vi "Create Pattern Script(Burst Length).vi"(8 "error in (no error)":errorcluster, 10 "BurstLength":T1, 11 "BML Pattern Creater in":refnum<class "BML Pattern Creater.lvclass">) -> (0 "error out":errorcluster, 2 "String":string, 3 "BML Pattern Creater out":refnum<class "BML Pattern Creater.lvclass">)   [LabVIEW 2018, in "BML Pattern Creater.lvlib" / "BML Pattern Creater.lvclass"]
uses:
  BML Pattern Creater.lvclass
  Ctls/Burst Length.ctl
  Interfaces/Protocol Interface.lvlibp/Interfaces/Protocol Interface/Pin State.ctl
  Interfaces/Protocol Interface.lvlibp/Interfaces/Protocol Interface/Protocol Interface.lvclass
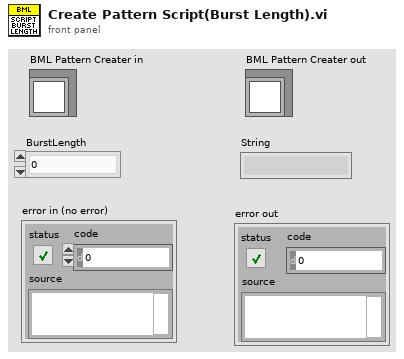
[diagram p1: front panel]
types:
  T1 = typedef "Burst Length.ctl" = enum8{"0", "2", "3", "4", "5", "8", "16", "32"}
  T2 = typedef "Protocol Interface.lvlibp/Protocol Interface.lvclass/Pin State.ctl" = enum16{"0", "1", "L", "H", "X", "V", "D", "M"}
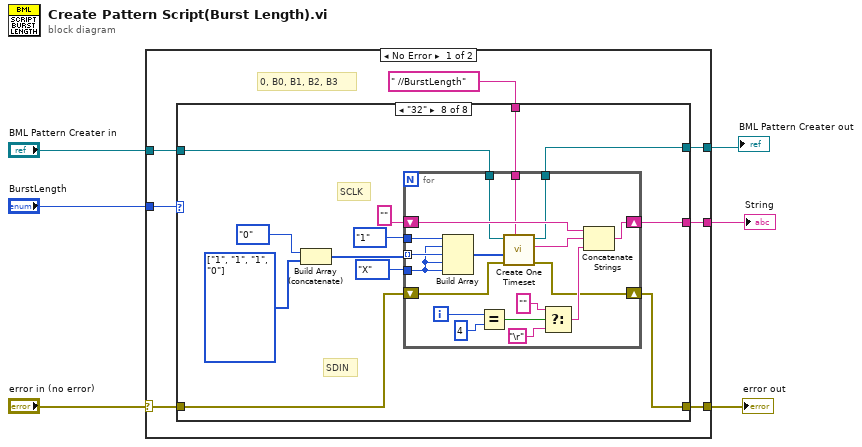
[diagram p0: block diagram]
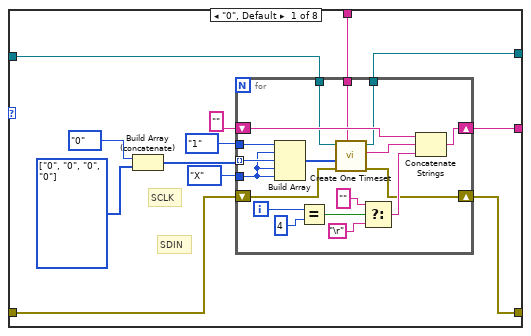
[diagram p2: hidden frame]
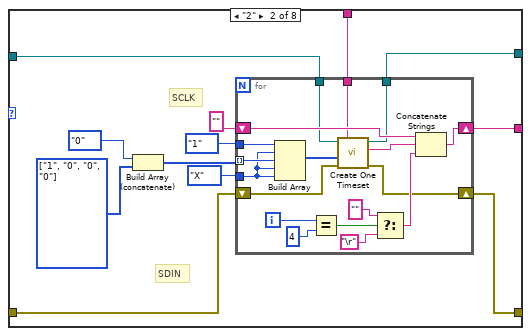
[diagram p3: hidden frame]
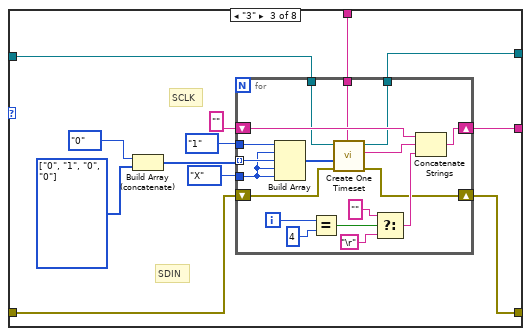
[diagram p4: hidden frame]
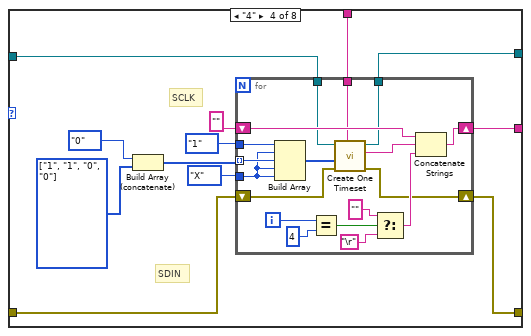
[diagram p5: hidden frame]
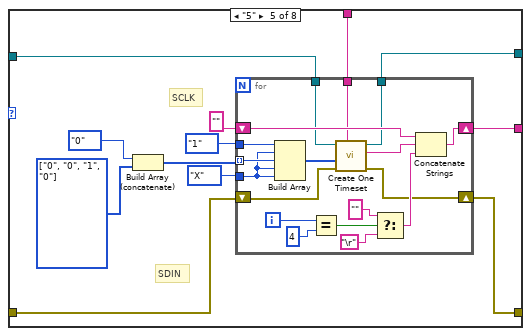
[diagram p6: hidden frame]
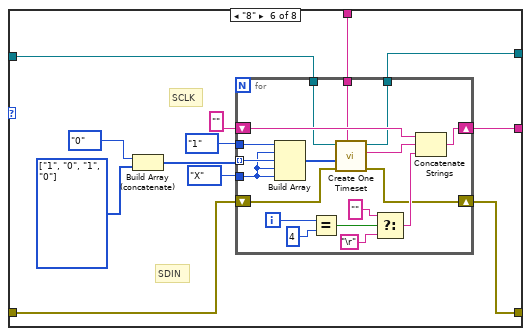
[diagram p7: hidden frame]
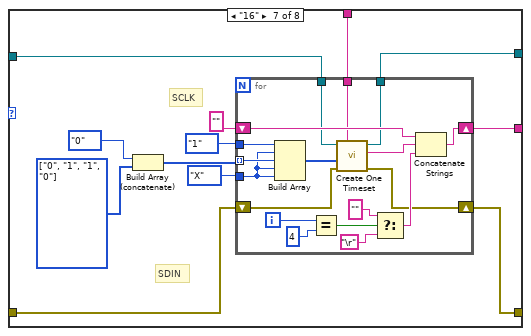
[diagram p8: hidden frame]
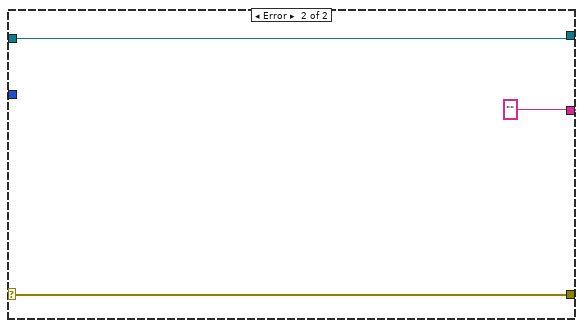
[diagram p9: hidden frame]
diagram:
  n1 = case shown="No Error" "error in (no error)" {
    selector: "error in (no error)" -> [w9 w255]
    tunnel: [w13 ""] -> w5
    tunnel: [w8 w255] -> w4
    tunnel: "BurstLength" -> [w11 _]
    tunnel: "BML Pattern Creater in" -> [w10 w254]
    tunnel: [w7 w254] -> w1
    frame No Error {
      # "0, B0, B1, B2, B3"
      n2 = case shown="\"32\"" w11 {
        tunnel: [w25 w55 w85 w115 w145 w175 w205 w235] -> w13
        tunnel: " //BurstLength" ("Notes") -> [w21 w51 w81 w111 w141 w171 w201 w231]
        tunnel: w10 -> [w17 w47 w77 w107 w137 w167 w197 w227]
        tunnel: [w16 w46 w76 w106 w136 w166 w196 w226] -> w7
        tunnel: w9 -> [w15 w45 w75 w105 w135 w165 w195 w225]
        tunnel: [w14 w44 w74 w104 w134 w164 w194 w224] -> w8
        frame "0", Default {
          w23 = T2[] [enum."0", enum."0", enum."0", enum."0"] items=["0", "1", "L", "H", "X", "V", "D", "M"] ("PinState")
          # "SCLK"
          # "SDIN"
          n3 = Build Array (concatenate)(Pin_State."0" ("PinState"), w23) -> (w22:T2[])
          n4 = for {
            tunnel: w22 -> [w34] mode=indexing
            shift-right: [w38] -> w25
            shift-left: "" -> [w37]
            tunnel: Pin_State."1" ("PinState") -> [w35]
            tunnel: Pin_State."X" ("PinState") -> [w33]
            tunnel: w21 -> [w32]
            tunnel: w17 -> [w29]
            tunnel: [w28] -> w16
            shift-right: [w26] -> w14
            shift-left: w15 -> [w27]
            i -> [w43]
            n5 = Build Array(w35, w33, w34, w33, w33) -> (w30:T2[])
            n6 = Equal?(x=w43, y=4) -> (x = y?=w41:bool)
            n7 = call-dynamic "Create One Timeset.vi"("Notes"=w32, "error in (no error)"=w27, "Pin State"=w30, "BML Pattern Creater in"=w29) -> ("error out"=w26:errorcluster, "string out"=w31:string, "BML Pattern Creater out"=w28:refnum<class "BML Pattern Creater.lvclass">)  [unwired: 5 in]
            n8 = Select(t="", s=w41, f="\r") -> (s? t:f=w36:string)
            n9 = Concatenate Strings(w37, w31, w36) -> (w38:string)
          }
        }
        frame "2" {
          w53 = T2[] [enum."1", enum."0", enum."0", enum."0"] items=["0", "1", "L", "H", "X", "V", "D", "M"] ("PinState")
          # "SCLK"
          # "SDIN"
          n10 = Build Array (concatenate)(Pin_State."0" ("PinState"), w53) -> (w52:T2[])
          n11 = for {
            tunnel: w52 -> [w64] mode=indexing
            shift-right: [w68] -> w55
            shift-left: "" -> [w67]
            tunnel: Pin_State."1" ("PinState") -> [w65]
            tunnel: Pin_State."X" ("PinState") -> [w63]
            tunnel: w51 -> [w62]
            tunnel: w47 -> [w59]
            tunnel: [w58] -> w46
            shift-right: [w56] -> w44
            shift-left: w45 -> [w57]
            i -> [w73]
            n12 = Build Array(w65, w63, w64, w63, w63) -> (w60:T2[])
            n13 = Equal?(x=w73, y=4) -> (x = y?=w71:bool)
            n14 = call-dynamic "Create One Timeset.vi"("Notes"=w62, "error in (no error)"=w57, "Pin State"=w60, "BML Pattern Creater in"=w59) -> ("error out"=w56:errorcluster, "string out"=w61:string, "BML Pattern Creater out"=w58:refnum<class "BML Pattern Creater.lvclass">)  [unwired: 5 in]
            n15 = Select(t="", s=w71, f="\r") -> (s? t:f=w66:string)
            n16 = Concatenate Strings(w67, w61, w66) -> (w68:string)
          }
        }
        frame "3" {
          w83 = T2[] [enum."0", enum."1", enum."0", enum."0"] items=["0", "1", "L", "H", "X", "V", "D", "M"] ("PinState")
          # "SCLK"
          # "SDIN"
          n17 = Build Array (concatenate)(Pin_State."0" ("PinState"), w83) -> (w82:T2[])
          n18 = for {
            tunnel: w82 -> [w94] mode=indexing
            shift-right: [w98] -> w85
            shift-left: "" -> [w97]
            tunnel: Pin_State."1" ("PinState") -> [w95]
            tunnel: Pin_State."X" ("PinState") -> [w93]
            tunnel: w81 -> [w90]
            tunnel: w77 -> [w89]
            tunnel: [w88] -> w76
            shift-right: [w86] -> w74
            shift-left: w75 -> [w87]
            i -> [w103]
            n19 = Build Array(w95, w93, w94, w93, w93) -> (w91:T2[])
            n20 = Equal?(x=w103, y=4) -> (x = y?=w101:bool)
            n21 = call-dynamic "Create One Timeset.vi"("Notes"=w90, "error in (no error)"=w87, "Pin State"=w91, "BML Pattern Creater in"=w89) -> ("error out"=w86:errorcluster, "string out"=w92:string, "BML Pattern Creater out"=w88:refnum<class "BML Pattern Creater.lvclass">)  [unwired: 5 in]
            n22 = Select(t="", s=w101, f="\r") -> (s? t:f=w96:string)
            n23 = Concatenate Strings(w97, w92, w96) -> (w98:string)
          }
        }
        frame "4" {
          w113 = T2[] [enum."1", enum."1", enum."0", enum."0"] items=["0", "1", "L", "H", "X", "V", "D", "M"] ("PinState")
          # "SCLK"
          # "SDIN"
          n24 = Build Array (concatenate)(Pin_State."0" ("PinState"), w113) -> (w112:T2[])
          n25 = for {
            tunnel: w112 -> [w124] mode=indexing
            shift-right: [w128] -> w115
            shift-left: "" -> [w127]
            tunnel: Pin_State."1" ("PinState") -> [w125]
            tunnel: Pin_State."X" ("PinState") -> [w123]
            tunnel: w111 -> [w122]
            tunnel: w107 -> [w120]
            tunnel: [w118] -> w106
            shift-right: [w116] -> w104
            shift-left: w105 -> [w117]
            i -> [w133]
            n26 = Build Array(w125, w123, w124, w123, w123) -> (w119:T2[])
            n27 = Equal?(x=w133, y=4) -> (x = y?=w131:bool)
            n28 = call-dynamic "Create One Timeset.vi"("Notes"=w122, "error in (no error)"=w117, "Pin State"=w119, "BML Pattern Creater in"=w120) -> ("error out"=w116:errorcluster, "string out"=w121:string, "BML Pattern Creater out"=w118:refnum<class "BML Pattern Creater.lvclass">)  [unwired: 5 in]
            n29 = Select(t="", s=w131, f="\r") -> (s? t:f=w126:string)
            n30 = Concatenate Strings(w127, w121, w126) -> (w128:string)
          }
        }
        frame "5" {
          w143 = T2[] [enum."0", enum."0", enum."1", enum."0"] items=["0", "1", "L", "H", "X", "V", "D", "M"] ("PinState")
          # "SCLK"
          # "SDIN"
          n31 = Build Array (concatenate)(Pin_State."0" ("PinState"), w143) -> (w142:T2[])
          n32 = for {
            tunnel: w142 -> [w154] mode=indexing
            shift-right: [w158] -> w145
            shift-left: "" -> [w157]
            tunnel: Pin_State."1" ("PinState") -> [w155]
            tunnel: Pin_State."X" ("PinState") -> [w153]
            tunnel: w141 -> [w152]
            tunnel: [w149] -> w136
            tunnel: w137 -> [w148]
            shift-right: [w146] -> w134
            shift-left: w135 -> [w147]
            i -> [w163]
            n33 = Build Array(w155, w153, w154, w153, w153) -> (w151:T2[])
            n34 = Equal?(x=w163, y=4) -> (x = y?=w161:bool)
            n35 = call-dynamic "Create One Timeset.vi"("Notes"=w152, "error in (no error)"=w147, "Pin State"=w151, "BML Pattern Creater in"=w148) -> ("error out"=w146:errorcluster, "string out"=w150:string, "BML Pattern Creater out"=w149:refnum<class "BML Pattern Creater.lvclass">)  [unwired: 5 in]
            n36 = Select(t="", s=w161, f="\r") -> (s? t:f=w156:string)
            n37 = Concatenate Strings(w157, w150, w156) -> (w158:string)
          }
        }
        frame "8" {
          w173 = T2[] [enum."1", enum."0", enum."1", enum."0"] items=["0", "1", "L", "H", "X", "V", "D", "M"] ("PinState")
          # "SCLK"
          # "SDIN"
          n38 = Build Array (concatenate)(Pin_State."0" ("PinState"), w173) -> (w172:T2[])
          n39 = for {
            tunnel: w172 -> [w184] mode=indexing
            shift-right: [w188] -> w175
            shift-left: "" -> [w187]
            tunnel: Pin_State."1" ("PinState") -> [w185]
            tunnel: Pin_State."X" ("PinState") -> [w183]
            tunnel: w171 -> [w182]
            tunnel: w167 -> [w179]
            tunnel: [w178] -> w166
            shift-right: [w176] -> w164
            shift-left: w165 -> [w177]
            i -> [w193]
            n40 = Build Array(w185, w183, w184, w183, w183) -> (w181:T2[])
            n41 = Equal?(x=w193, y=4) -> (x = y?=w191:bool)
            n42 = call-dynamic "Create One Timeset.vi"("Notes"=w182, "error in (no error)"=w177, "Pin State"=w181, "BML Pattern Creater in"=w179) -> ("error out"=w176:errorcluster, "string out"=w180:string, "BML Pattern Creater out"=w178:refnum<class "BML Pattern Creater.lvclass">)  [unwired: 5 in]
            n43 = Select(t="", s=w191, f="\r") -> (s? t:f=w186:string)
            n44 = Concatenate Strings(w187, w180, w186) -> (w188:string)
          }
        }
        frame "16" {
          w203 = T2[] [enum."0", enum."1", enum."1", enum."0"] items=["0", "1", "L", "H", "X", "V", "D", "M"] ("PinState")
          # "SCLK"
          # "SDIN"
          n45 = Build Array (concatenate)(Pin_State."0" ("PinState"), w203) -> (w202:T2[])
          n46 = for {
            tunnel: w202 -> [w214] mode=indexing
            shift-right: [w218] -> w205
            shift-left: "" -> [w217]
            tunnel: Pin_State."1" ("PinState") -> [w215]
            tunnel: Pin_State."X" ("PinState") -> [w213]
            tunnel: w201 -> [w212]
            tunnel: w197 -> [w209]
            tunnel: [w208] -> w196
            shift-right: [w206] -> w194
            shift-left: w195 -> [w207]
            i -> [w223]
            n47 = Build Array(w215, w213, w214, w213, w213) -> (w211:T2[])
            n48 = Equal?(x=w223, y=4) -> (x = y?=w221:bool)
            n49 = call-dynamic "Create One Timeset.vi"("Notes"=w212, "error in (no error)"=w207, "Pin State"=w211, "BML Pattern Creater in"=w209) -> ("error out"=w206:errorcluster, "string out"=w210:string, "BML Pattern Creater out"=w208:refnum<class "BML Pattern Creater.lvclass">)  [unwired: 5 in]
            n50 = Select(t="", s=w221, f="\r") -> (s? t:f=w216:string)
            n51 = Concatenate Strings(w217, w210, w216) -> (w218:string)
          }
        }
        frame "32" {
          w233 = T2[] [enum."1", enum."1", enum."1", enum."0"] items=["0", "1", "L", "H", "X", "V", "D", "M"] ("PinState")
          # "SCLK"
          # "SDIN"
          n52 = Build Array (concatenate)(Pin_State."0" ("PinState"), w233) -> (w232:T2[])
          n53 = for {
            tunnel: w232 -> [w244] mode=indexing
            shift-right: [w248] -> w235
            shift-left: "" -> [w247]
            tunnel: Pin_State."1" ("PinState") -> [w245]
            tunnel: Pin_State."X" ("PinState") -> [w243]
            tunnel: w231 -> [w242]
            tunnel: w227 -> [w239]
            tunnel: [w238] -> w226
            shift-right: [w236] -> w224
            shift-left: w225 -> [w237]
            i -> [w253]
            n54 = Build Array(w245, w243, w244, w243, w243) -> (w240:T2[])
            n55 = Equal?(x=w253, y=4) -> (x = y?=w251:bool)
            n56 = call-dynamic "Create One Timeset.vi"("Notes"=w242, "error in (no error)"=w237, "Pin State"=w240, "BML Pattern Creater in"=w239) -> ("error out"=w236:errorcluster, "string out"=w241:string, "BML Pattern Creater out"=w238:refnum<class "BML Pattern Creater.lvclass">)  [unwired: 5 in]
            n57 = Select(t="", s=w251, f="\r") -> (s? t:f=w246:string)
            n58 = Concatenate Strings(w247, w241, w246) -> (w248:string)
          }
        }
      }
    }
    frame Error {
    }
  }
  "String" <- w5
  "error out" <- w4
  "BML Pattern Creater out" <- w1
